vi "Arret Urgence.vi"() -> (0 "error out":errorcluster)   [LabVIEW 2014]
panel:
  in  "error in (no error)":errorcluster
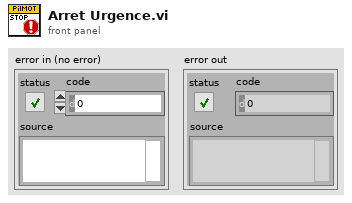
[diagram p1: front panel]
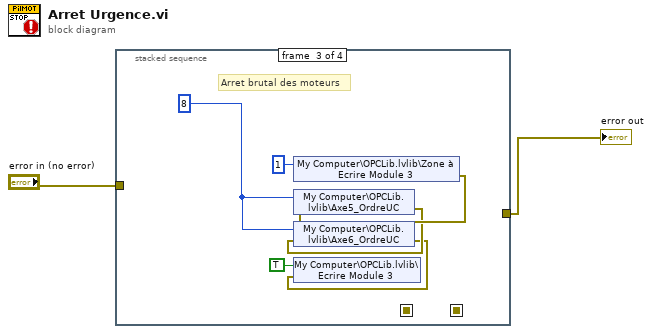
[diagram p0: block diagram]
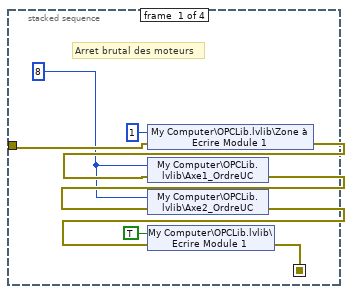
[diagram p2: hidden frame]
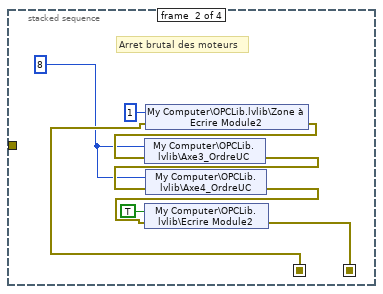
[diagram p3: hidden frame]
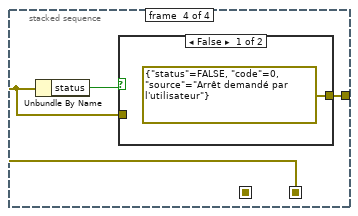
[diagram p4: hidden frame]
diagram:
  n1 = stacked-sequence {
    seq-local: [_ w14 _ _] -> [_ _ _ w25]
    seq-local: [w5 _ _ _] -> [_ w13 _ _]
    tunnel: "error in (no error)" -> [w9 _ _ _]
    tunnel: [_ _ _ w26] -> w1
    frame #0 {
      w4 = u16 8 ("Axe1_OrdreUC")
      # "Arret brutal des moteurs"
      n2 = shared-variable "My Computer\\OPCLib.lvlib\\Zone à Ecrire Module 1"(u16 1 ("Zone à Ecrire Module 1"), error in=w9) -> (error out=w8:errorcluster)
      n3 = shared-variable "My Computer\\OPCLib.lvlib\\Axe1_OrdreUC"(w4, error in=w8) -> (error out=w7:errorcluster)
      n4 = shared-variable "My Computer\\OPCLib.lvlib\\Axe2_OrdreUC"(w4, error in=w7) -> (error out=w6:errorcluster)
      n5 = shared-variable "My Computer\\OPCLib.lvlib\\Ecrire Module 1"(TRUE ("Ecrire Module 1"), error in=w6) -> (error out=w5:errorcluster)
    }
    frame #1 {
      w12 = u16 8 ("Axe3_OrdreUC")
      # "Arret brutal des moteurs"
      n6 = shared-variable "My Computer\\OPCLib.lvlib\\Zone à Ecrire Module2"(u16 1 ("Zone à Ecrire Module2"), error in=w13) -> (error out=w17:errorcluster)
      n7 = shared-variable "My Computer\\OPCLib.lvlib\\Axe3_OrdreUC"(w12, error in=w17) -> (error out=w16:errorcluster)
      n8 = shared-variable "My Computer\\OPCLib.lvlib\\Axe4_OrdreUC"(w12, error in=w16) -> (error out=w15:errorcluster)
      n9 = shared-variable "My Computer\\OPCLib.lvlib\\Ecrire Module2"(TRUE ("Ecrire Module2"), error in=w15) -> (error out=w14:errorcluster)
    }
    frame #2 {
      w23 = u16 8 ("Axe1_OrdreUC")
      # "Arret brutal des moteurs"
      n10 = shared-variable "My Computer\\OPCLib.lvlib\\Zone à Ecrire Module 3"(u16 1 ("Zone à Ecrire Module 1")) -> (error out=w21:errorcluster)  [unwired: 1 in]
      n11 = shared-variable "My Computer\\OPCLib.lvlib\\Axe5_OrdreUC"(w23, error in=w21) -> (error out=w20:errorcluster)
      n12 = shared-variable "My Computer\\OPCLib.lvlib\\Axe6_OrdreUC"(w23, error in=w20) -> (error out=w19:errorcluster)
      n13 = shared-variable "My Computer\\OPCLib.lvlib\\Ecrire Module 3"(TRUE ("Ecrire Module 1"), error in=w19) -> ()  [unwired: 1 out]
    }
    frame #3 {
      n14 = Unbundle By Name(w25) -> ("status"=w27:bool)
      n15 = case shown="False" w27 {
        tunnel: [errorcluster {"status"=FALSE, "code"=0, "source"="Arrêt demandé par l'utilisateur"} ("error out") w29] -> w26
        tunnel: w25 -> [_ w29]
        frame False {
        }
        frame True {
        }
      }
    }
  }
  "error out" <- w1
